vi "Generate Channel Numbers.vi"(8 "error in (no error)":errorcluster, 9 "Index":i32) -> (0 "error out":errorcluster, 1 "Number":string)   [LabVIEW 2017]
doc: "If 0<Index <9 then Add char '0\"\nelse just put in a value through"
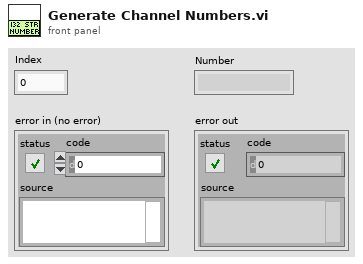
[diagram p1: front panel]
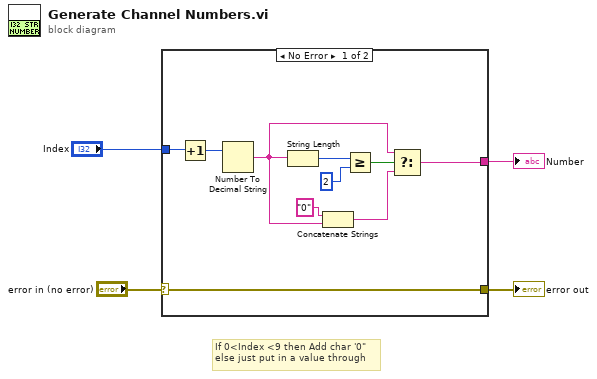
[diagram p0: block diagram]
diagram:
  # "If 0<Index <9 then Add char '0\"\nelse just put in a value through"
  n1 = case shown="No Error" "error in (no error)" {
    selector: "error in (no error)" -> [w14 w15]
    tunnel: [w14 w15] -> w3
    tunnel: "Index" -> [w6 _]
    tunnel: [w7 _] -> w1
    frame No Error {
      n2 = Increment(x=w6) -> (x+1=w5:i32)
      n3 = Number To Decimal String(number=w5) -> (decimal integer string=w9:string)  [unwired: 1 in]
      n4 = String Length(string=w9) -> (length=w13:i32)
      n5 = Concatenate Strings("0" ("string"), w9) -> (w8:string)
      n6 = Greater Or Equal?(x=w13, y=2) -> (x >= y?=w11:bool)
      n7 = Select(t=w9, s=w11, f=w8) -> (s? t:f=w7:string)
    }
    frame Error {
    }
  }
  "error out" <- w3
  "Number" <- w1
